vi "Glimpse sequence player compute next frame number.vi"(4 "Current Frame Number":u32, 5 "Loop?":bool, 6 "# of Frames in sequence/FOV":u32, 7 "Current Mode":enum16{"Stop", "Play Forward", "Play Backward"}(ring), 8 "Range In":cluster{"Max":u32, "Min":u32}, 9 "Range Enabled":bool) -> (0 "Current Frame Number Out":u32, 1 "Current Mode Out":enum16{"Stop", "Play Forward", "Play Backward"}(ring), 2 "Range Out":cluster{"Max":u32, "Min":u32})   [LabVIEW 2016]
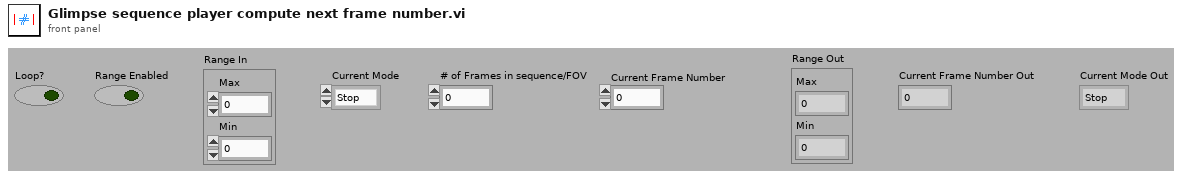
[diagram p1: front panel]
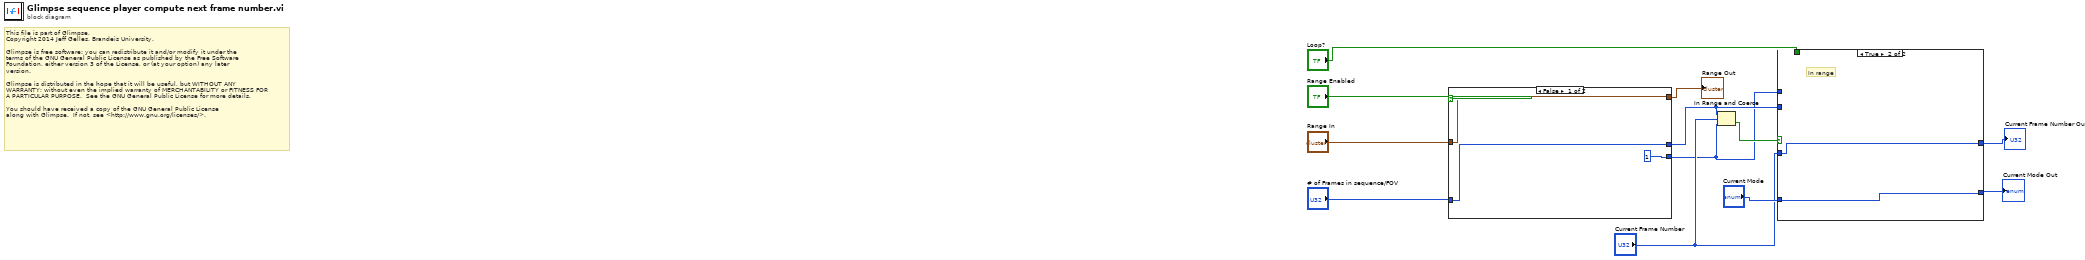
[diagram p0: block diagram]
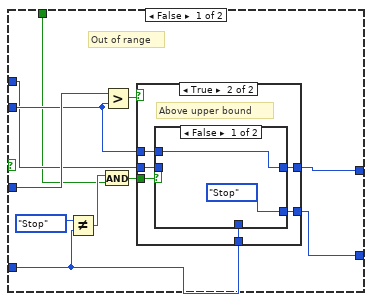
[diagram p2: hidden frame]
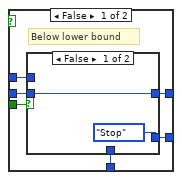
[diagram p3: hidden frame]
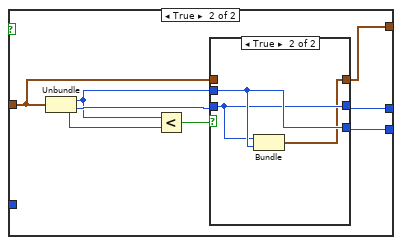
[diagram p6: hidden frame]
diagram:
  # "This file is part of Glimpse. \nCopyright 2014 Jeff Gelles, Brandeis University.    \n\nGlimpse is free software: you can redistribute it and/or modify it under the \nterms of the GNU General Public License as published by the Free Software \nFoundation, either version 3 of the License, or (at your option) any later \nversion.\n\nGlimpse is distributed in the hope that it will be useful, but WITHOUT ANY \nWARRANTY; without even the implied warranty of MERCHANTABILITY or FITNESS FOR \nA PARTICULAR PURPOSE.  See the GNU General Public License for more details.\n\nYou should have received a copy of the GNU General Public License\nalong with Glimpse.  If not, see <http://www.gnu.org/licenses/>."
  n1 = case shown="False" "Range Enabled" {
    tunnel: [i16 1 w18] -> w6
    tunnel: [w15 w19] -> w7
    tunnel: "# of Frames in sequence/FOV" -> [w15 _]
    tunnel: "Range In" -> [w13 w16]
    tunnel: [w13 w17] -> w12
    frame False {
    }
    frame True {
      n2 = Unbundle(w16) -> ("Max"=w20:u32, "Min"=w21:u32)
      n3 = Less?(x=w20, y=w21) -> (x < y?=w22:bool)
      n4 = case shown="True" w22 {
        tunnel: w21 -> [w24 w27]
        tunnel: w20 -> [w25 w28]
        tunnel: [w25 w27] -> w19
        tunnel: [w24 w28] -> w18
        tunnel: [w23 w26] -> w17
        tunnel: w16 -> [w23 _]
        frame False {
        }
        frame True {
          n5 = Bundle("Min"=w27, "Max"=w28) -> (w26:cluster{"Min":u32, "Max":u32})  [unwired: 1 out]
        }
      }
    }
  }
  "Range Out" <- w12
  n6 = In Range and Coerce(upper limit=w7, x="Current Frame Number", lower limit=w6) -> (In Range?=w8:bool)  [unwired: 1 out]
  n7 = case shown="True" w8 {
    tunnel: w6 -> [w34 _]
    tunnel: w7 -> [w35 _]
    tunnel: "Current Frame Number" -> [w39 w61]
    tunnel: [w37 w61] -> w2
    tunnel: [w36 w60] -> w1
    tunnel: "Current Mode" -> [w30 w60]
    tunnel: "Loop?" -> [w29 _]
    frame False {
      # "Out of range"
      n8 = Not Equal?(x=enum16{"Stop", "Play Forward", "Play Backward"}."Stop", y=w30) -> (x != y?=w32:bool)
      n9 = And(x=w32, y=w29) -> (x .and. y?=w33:bool)
      n10 = Greater?(x=w39, y=w35) -> (0:w38:bool)
      n11 = case shown="True" w38 {
        tunnel: w33 -> [w45 w55]
        tunnel: w34 -> [w44 w54]
        tunnel: [w43 w53] -> w37
        tunnel: [w42 w52] -> w36
        tunnel: w35 -> [w41 w51]
        tunnel: w30 -> [w40 w50]
        frame False {
          # "Below lower bound"
          n12 = case shown="False" w45 {
            tunnel: w44 -> [w47 _]
            tunnel: [w47 w49] -> w43
            tunnel: [enum16{"Stop", "Play Forward", "Play Backward"}."Stop" ("Current Mode") w48] -> w42
            tunnel: w41 -> [_ w49]
            tunnel: w40 -> [_ w48]
            frame False {
            }
            frame True {
            }
          }
        }
        frame True {
          # "Above upper bound"
          n13 = case shown="False" w55 {
            tunnel: w54 -> [_ w59]
            tunnel: [w57 w59] -> w53
            tunnel: [enum16{"Stop", "Play Forward", "Play Backward"}."Stop" ("Current Mode") w58] -> w52
            tunnel: w51 -> [w57 _]
            tunnel: w50 -> [_ w58]
            frame False {
            }
            frame True {
            }
          }
        }
      }
    }
    frame True {
      # "In range"
    }
  }
  "Current Frame Number Out" <- w2
  "Current Mode Out" <- w1
